vi "Get Database Info.vi"(11 "2D Array in":string[][](array[string])) -> (1 "Array":u32[](array[numeric]), 3 "2D Array in 2":string[](array[string]))   [LabVIEW 2014]
doc: "This SubVI gets the database (a CSV file), which is typically a 2D array, and returns a 1D array of components. It also provides a 1D array of number of components per category."
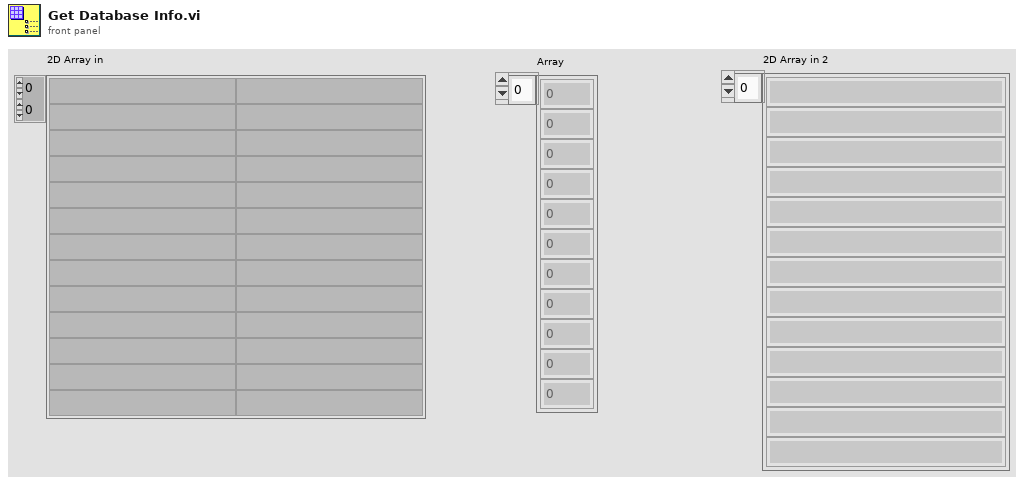
[diagram p1: front panel]
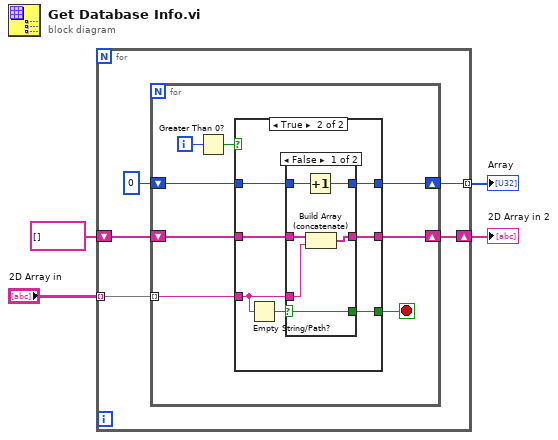
[diagram p0: block diagram]
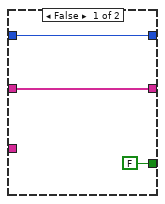
[diagram p2: hidden frame]
diagram:
  n1 = for {
    tunnel: "2D Array in" -> [w9] mode=indexing
    shift-right: [w7] -> w3
    shift-left: string[] [] ("2D Array in") -> [w8]
    tunnel: [w5] -> w2 mode=indexing
    n2 = for {
      tunnel: w9 -> [w15] mode=indexing
      shift-right: [w13] -> w7
      shift-left: w8 -> [w14]
      shift-right: [w11] -> w5
      shift-left: u32 0 -> [w12]
      i -> [w17]
      stop <- w10 stop-if-true
      n3 = Greater Than 0?(x=w17) -> (x > 0?=w16:bool)
      n4 = case shown="True" w16 {
        tunnel: w15 -> [_ w24]
        tunnel: w14 -> [w20 w25]
        tunnel: [w20 w26] -> w13
        tunnel: w12 -> [w19 w23]
        tunnel: [w19 w22] -> w11
        tunnel: [FALSE w21] -> w10
        frame False {
        }
        frame True {
          n5 = Empty String/Path?(string/path=w24) -> (empty?=w27:bool)
          n6 = case shown="False" w27 {
            selector: w27 -> [w28 w34]
            tunnel: [w31 w36] -> w26
            tunnel: w25 -> [w32 w36]
            tunnel: w24 -> [w33 _]
            tunnel: w23 -> [w30 w35]
            tunnel: [w29 w35] -> w22
            tunnel: [w28 w34] -> w21
            frame False {
              n7 = Increment(x=w30) -> (x+1=w29:u32)
              n8 = Build Array (concatenate)(w32, w33) -> (w31:string[])
            }
            frame True {
            }
          }
        }
      }
    }
  }
  "2D Array in 2" <- w3
  "Array" <- w2
